vi "niRFUtil RFHS Util Dll Path.vi"() -> (0 "Library version":u32 format="%08x", 1 "Library info":string, 2 "error out":errorcluster, 3 "Path":path, 4 "AVX support":bool)   [LabVIEW 2015, in "niRFUtil.lvlib"]
uses:
  niRFUtil.lvlib
  <vilib>/Utility/sysdir.llb/System Directory Type.ctl
  Channelizer/Includes/niRFUtil RFHS Channelizer ChannelizerErrors.ctl
panel:
  out "Library version":string
  in  "Additional search path":path[](array[path])=[path "m:/RfProtocols/RFmx/DLLs/niRFHS/trunk/2.1/dist/win64U", path "m:/RfProtocols/RFmx/DLLs/niRFHS/trunk/2.1/dist/win32U"]
  # "Search order:\n1) system folder (e.g. c:\\windows\\system32)\n2) r:\\\n3) additional search paths given above"
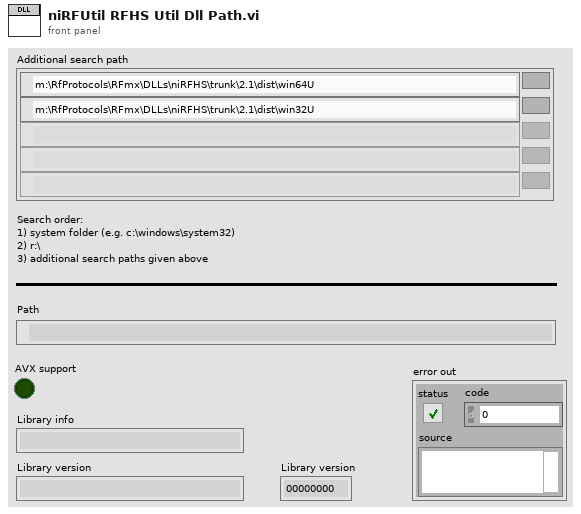
[diagram p1: front panel]
types:
  T1 = typedef "niRFUtil.lvlib/niRFUtil RFHS Channelizer ChannelizerErrors.ctl" = enum32{"No Error", "Invalid Channel", "Internal Error", "Invalid Channel fs", "Invalid Phase Shift", "Invalid fs", "Invalid Number Of Channles", "Invalid FFT Channel fs", "Invalid Resampler Channel fs", "Not a 15kHz Multiple", "Invalid Channel fc", "Invalid passBW/stopBW", "Coerced Rejection", "Requires Internal Buffer", "Duplicated Destination Channel Name", "Configuration Format Error", "Illegal Execution state", "DLL not found", "DLL loading failure", "AVX instruction failure"}
  T2 = typedef "System Directory Type.ctl" = i32
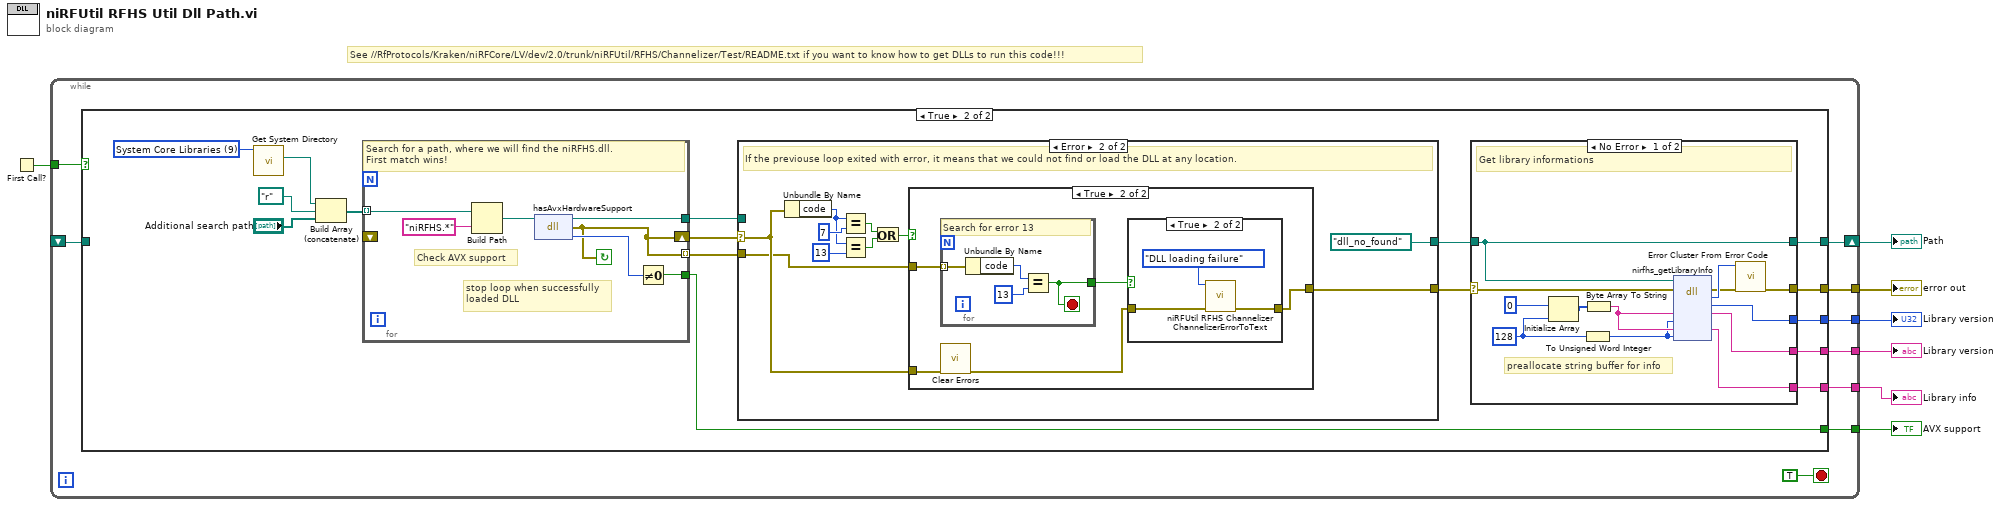
[diagram p0: block diagram]
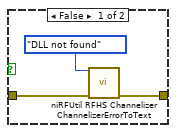
[diagram p6: hidden frame]
diagram:
  # "See //RfProtocols/Kraken/niRFCore/LV/dev/2.0/trunk/niRFUtil/RFHS/Channelizer/Test/README.txt if you want to know how to get DLLs to run this code!!!"
  n1 = First Call?() -> (First Call?: T/F=w7:bool)
  n2 = while {
    tunnel: w7 -> [w14]
    shift-right: [w15] -> w2
    shift-left: _ -> [w12]
    tunnel: [w13] -> w6
    tunnel: [w11] -> w5
    tunnel: [w10] -> w4
    tunnel: [w9] -> w3
    tunnel: [w8] -> w1
    stop <- TRUE stop-if-true
    n3 = case shown="True" w14 {
      tunnel: [w17 w28] -> w15
      tunnel: [_ w30] -> w13
      tunnel: w12 -> [w17 _]
      tunnel: [_ w19] -> w11
      tunnel: [_ w27] -> w10
      tunnel: [_ w26] -> w9
      tunnel: [_ w25] -> w8
      frame False {
        # "This case is executed on al non-intitial executions of this vi. \nIt will use the values computed at the first execution. This\navoids the expensive DLL detection the be executed over \nand over again."
      }
      frame True {
        w33 = T2 9 items=["User Home"=0, "User Desktop"=1, "User Documents"=2, "User Application Data"=3, "User Preferences"=4, "User Temporary"=5, "Public Documents"=6, "Public Application Data"=7, "Public Preferences"=8, "Public Cache"=13, "System Core Libraries"=9, "System Installed Libraries"=10, "Application Files"=11, "Boot Volume Root"=12] ("system directory type")
        n4 = call <vilib>:"Get System Directory.vi"("system directory type"=w33) -> ("system directory"=w32:path)  [unwired: 10 in]
        n5 = Build Array (concatenate)(w32, path "r:/" ("system directory"), "Additional search path") -> (w22:path[])
        n6 = for {
          tunnel: w22 -> [w52] mode=indexing
          shift-right: [w49] -> w21
          shift-left: _ -> [_]
          tunnel: [w53] -> w18
          tunnel: [w50] -> w19
          tunnel: [w49] -> w20 mode=indexing
          stop <- w49 continue-if-true
          # "stop loop when successfully\nloaded DLL"
          # "Check AVX support"
          # "Search for a path, where we will find the niRFHS.dll. \nFirst match wins!"
          n7 = Build Path(base path=w52, name or relative path="niRFHS.*") -> (appended path=w54:path)
          n8 = dll-call lib="M:/RfProtocols/RFmx/DLLs/niRFHS/trunk/2.0/dist/win32U/niRFHS_generic.*" fn="hasAvxHardwareSupport"(path in=w54) -> (path out=w53:path, error out=w49:errorcluster, "return type"=w51:i32)  [unwired: 2 in]
          n9 = Not Equal To 0?(x=w51) -> (x != 0?=w50:bool)
        }
        n10 = case shown="Error" w21 {
          selector: w21 -> [w57 w65]
          tunnel: [w57 w64] -> w31
          tunnel: [w56 path "dll_no_found" ("Path")] -> w29
          tunnel: w18 -> [w56 _]
          tunnel: w20 -> [_ w63]
          frame No Error {
            # "check for a AVX capable library, that is executable."
          }
          frame Error {
            # "If the previouse loop exited with error, it means that we could not find or load the DLL at any location."
            n11 = Unbundle By Name(w65) -> ("code"=w61:i32)
            n12 = Equal?(x=w61, y=7) -> (x = y?=w62:bool)
            n13 = Equal?(x=w61, y=13) -> (x = y?=w58:bool)
            n14 = Or(x=w62, y=w58) -> (x .or. y?=w59:bool)
            n15 = case shown="True" w59 {
              tunnel: w65 -> [w68 w71]
              tunnel: [w68 w73] -> w64
              tunnel: w63 -> [_ w72]
              frame False {
              }
              frame True {
                n16 = for {
                  tunnel: w72 -> [w83] mode=indexing
                  tunnel: [w80] -> w70
                  stop <- w80 stop-if-true
                  # "Search for error 13"
                  n17 = Unbundle By Name(w83) -> ("code"=w82:i32)
                  n18 = Equal?(x=w82, y=13) -> (x = y?=w80:bool)
                }
                n19 = call <vilib>:"Clear Errors.vi"("error in (no error)"=w71) -> ("error out"=w69:errorcluster)  [unwired: 5 in, 1 out]
                n20 = case shown="True" w70 {
                  tunnel: [w76 w79] -> w73
                  tunnel: w69 -> [w74 w77]
                  frame False {
                    n21 = call "niRFUtil RFHS Channelizer ChannelizerErrorToText.vi"("Error List"=niRFUtil_RFHS_Channelizer_ChannelizerErrors."DLL not found", "error in (no error)"=w74) -> ("error out"=w76:errorcluster)  [unwired: 13 in]
                  }
                  frame True {
                    n22 = call "niRFUtil RFHS Channelizer ChannelizerErrorToText.vi"("Error List"=niRFUtil_RFHS_Channelizer_ChannelizerErrors."DLL loading failure", "error in (no error)"=w77) -> ("error out"=w79:errorcluster)  [unwired: 13 in]
                  }
                }
              }
            }
          }
        }
        n23 = case shown="No Error" w31 {
          selector: w31 -> [w46 w48]
          tunnel: [w43 w48] -> w30
          tunnel: [w40 _] -> w27
          tunnel: [w39 _] -> w26
          tunnel: w29 -> [w38 w47]
          tunnel: [w38 w47] -> w28
          tunnel: [w34 _] -> w25
          frame No Error {
            w36 = 128 ("dimension size")
            # "preallocate string buffer for info"
            # "Get library informations"
            n24 = Initialize Array(u8 0 ("element"), w36) -> (w41:u8[])
            n25 = To Unsigned Word Integer(number=w36) -> (unsigned 16bit integer=w35:u16)
            n26 = Byte Array To String(unsigned byte array=w41) -> (string=w37:string)
            n27 = dll-call lib="M:/RfProtocols/RFmx/DLLs/niRFHS/trunk/2.0/dist/win32U/niRFHS_generic.*" fn="nirfhs_getLibraryInfo"(path in=w38, error in=w46, "versionString"=w37, "versionStringBufSize"=w35, "info"=w37, "infoBufSize"=w35) -> (error out=w44:errorcluster, "return type"=w45:i32, "version"=w40:u32, "versionString"=w34:string, "info"=w39:string)  [unwired: 4 in, 1 out]
            n28 = call <vilib>:"Error Cluster From Error Code.vi"("error in (no error)"=w44, "error code (0)"=w45) -> ("error out"=w43:errorcluster)  [unwired: 7 in]
          }
          frame Error {
          }
        }
      }
    }
  }
  "Path" <- w2
  "error out" <- w6
  "AVX support" <- w5
  "Library version" <- w4
  "Library info" <- w3
  "Library version" <- w1
